vi "fastdaq.vi"() -> ()   [LabVIEW 2020]
uses:
  <vilib>/DAQmx/read.llb/DAQmx Read (Analog Wfm 1Chan NSamp).vi
  <vilib>/DAQmx/create/channels.llb/DAQmx Create Channel (AI-Voltage-Basic).vi
  <vilib>/DAQmx/configure/timing.llb/DAQmx Timing (Sample Clock).vi
  <vilib>/DAQmx/miscellaneous.llb/DAQmx Fill In Error Info.vi
  <resource>/objmgr/daqmx.rc
panel:
  in  "stop":bool
  out "Numeric":dbl
  out "Waveform Graph":waveform(dbl)(graph)
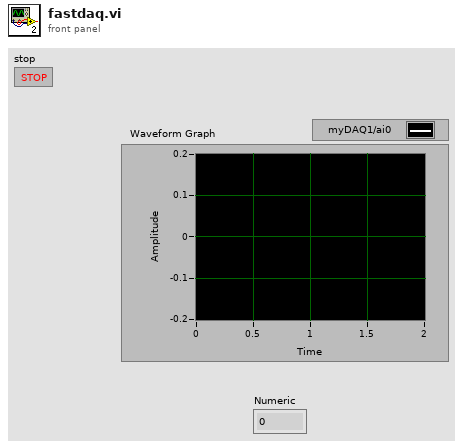
[diagram p1: front panel]
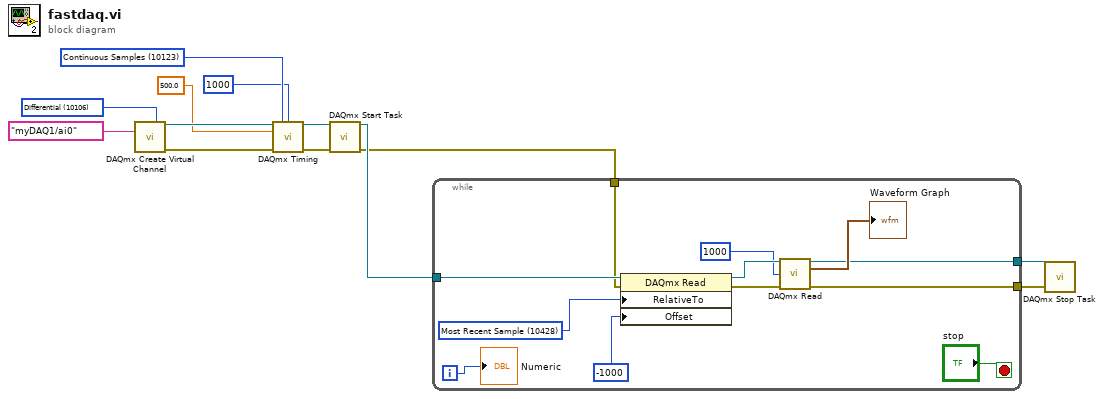
[diagram p0: block diagram]
diagram:
  w8 = 10123 items=["Finite Samples"=10178, "Continuous Samples"=10123, "Hardware Timed Single Point"=12522] ("sample mode")
  w10 = 10106 items=["Default"=-1, "RSE"=10083, "NRSE"=10078, "Differential"=10106, "Pseudodifferential"=12529] ("input terminal configuration")
  n1 = call-poly <vilib>:"DAQmx Create Virtual Channel.vi"("input terminal configuration"=w10, "physical channels"=tag "myDAQ1/ai0") -> ("task out"=w12:refnum<k21>, "error out"=w11:errorcluster)  [unwired: 12 in]
  n2 = call-poly <vilib>:"DAQmx Timing.vi"("task/channels in"=w12, "sample mode"=w8, "samples per channel"=1000, "rate"=500.0, "error in"=w11) -> ("task out"=w6:refnum<k21>, "error out"=w5:errorcluster)  [unwired: 9 in]
  n3 = call <vilib>:"DAQmx Start Task.vi"("task/channels in"=w6, "error in"=w5) -> ("task out"=w4:refnum<k21>, "error out"=w3:errorcluster)  [unwired: 12 in]
  n4 = while {
    tunnel: w4 -> [w21]
    tunnel: w3 -> [w20]
    tunnel: [w17] -> w2
    tunnel: [w16] -> w1
    i -> [w14]
    stop <- "stop" stop-if-true
    w19 = 10428 items=["First Sample"=10424, "Current Read Position"=10425, "Reference Trigger"=10426, "First Pretrigger Sample"=10427, "Most Recent Sample"=10428] ("RelativeTo")
    n5 = property class="DAQmx Read"(reference=w21, error in=w20, "RelativeTo"=w19, "Offset"=-1000) -> (reference out=w23:refnum<k21>, error out=w24:errorcluster)
    n6 = call-poly <vilib>:"DAQmx Read.vi"("task/channels in"=w23, "number of samples per channel"=1000, "error in"=w24) -> ("task out"=w17:refnum<k21>, "data"=→"Waveform Graph":waveform(dbl), "error out"=w16:errorcluster)  [unwired: 10 in]
    "Numeric" <- w14
  }
  n7 = call <vilib>:"DAQmx Stop Task.vi"("task/channels in"=w2, "error in"=w1) -> ()  [unwired: 12 in, 2 out]
